vi "CPU_MEM_CIA 1.vi"(5 "read all":bool, 7 "oper":enum16{"init", "read", "write"}(ring), 10 "value in":u8 format="%02x", 11 "address":u16 format="%04x") -> (2 "value out":u8 format="%02x", 3 "mem":u8[](array[numeric])=[27, 8, 14, 6, 20] format="%02x")   [LabVIEW 2018]
uses:
  CIA/CIA_IRQ_oper.ctl
  CIA/CIA1/CIA1_glb.vi
panel:
  in  "init size":u16=255 format="%.0x"
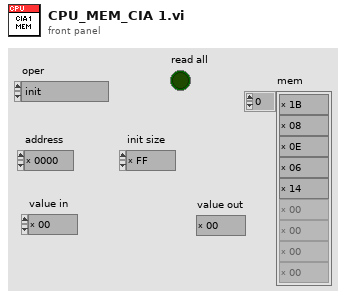
[diagram p1: front panel]
types:
  T1 = typedef "CIA_IRQ_oper.ctl" = enum16{"init", "set mask", "set flag", "check active", "read reg"}
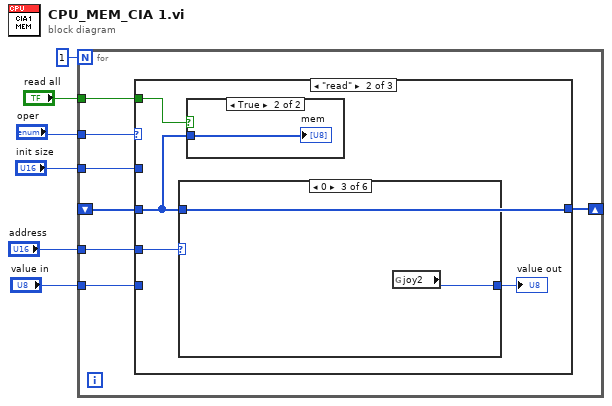
[diagram p0: block diagram]
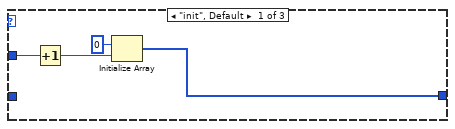
[diagram p2: hidden frame]
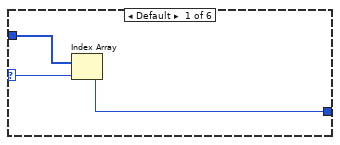
[diagram p4: hidden frame]
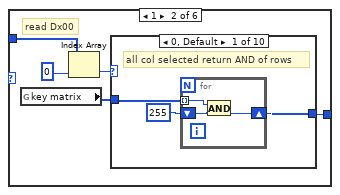
[diagram p5: hidden frame]
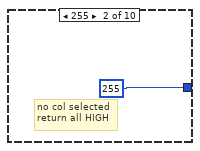
[diagram p6: hidden frame]
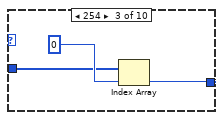
[diagram p7: hidden frame]
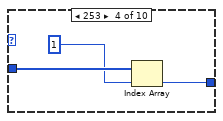
[diagram p8: hidden frame]
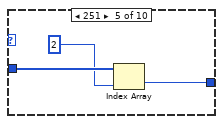
[diagram p9: hidden frame]
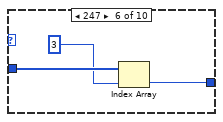
[diagram p10: hidden frame]
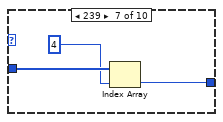
[diagram p11: hidden frame]
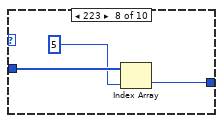
[diagram p12: hidden frame]
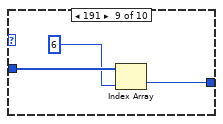
[diagram p13: hidden frame]
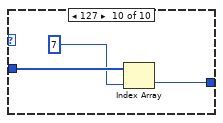
[diagram p14: hidden frame]
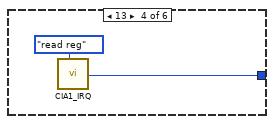
[diagram p15: hidden frame]
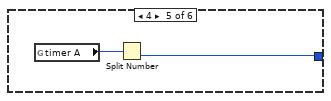
[diagram p16: hidden frame]
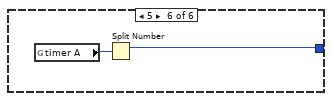
[diagram p17: hidden frame]
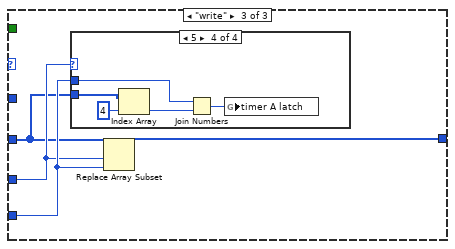
[diagram p18: hidden frame]
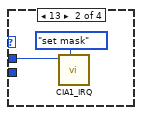
[diagram p20: hidden frame]
diagram:
  n1 = for {
    N: 1 -> [_]
    shift-right: [w11] -> _
    shift-left: _ -> [w10]
    tunnel: "oper" -> [w13]
    tunnel: "init size" -> [w12]
    tunnel: "address" -> [w9]
    tunnel: "value in" -> [w8]
    tunnel: "read all" -> [w7]
    n2 = case shown="\"read\"" w13 {
      tunnel: w12 -> [w17 _ _]
      tunnel: [w14 w19 w71] -> w11
      tunnel: w10 -> [_ w19 w69]
      tunnel: w9 -> [_ w21 w70]
      tunnel: w8 -> [_ _ w72]
      tunnel: w7 -> [_ w20 _]
      frame "init", Default {
        n3 = Increment(x=w17) -> (x+1=w15:u16)
        n4 = Initialize Array(u8 0 ("element"), w15) -> (w14:u8[])
      }
      frame "read" {
        n5 = case shown="0" w21 {
          selector: w21 -> [w23 _ _ _ _ _]
          tunnel: w19 -> [w25 w29 _ _ _ _]
          tunnel: [w24 w26 w62 w63 w65 w67] -> w18
          frame Default {
            n6 = Index Array(array=w25, index=w23) -> (element=w24:u8)
          }
          frame 1 {
            # "read Dx00"
            n7 = global read "CIA1_glb.vi" "key matrix"() -> (w30:u8[])
            n8 = Index Array(array=w29, index=0) -> (element=w28:u8)
            n9 = case shown="0, Default" w28 {
              tunnel: w30 -> [w33 _ w39 w43 w46 w49 w52 w55 w58 w61]
              tunnel: [w32 u8 255 ("y") w38 w41 w44 w47 w50 w53 w56 w59] -> w26
              frame 0, Default {
                # "all col selected return AND of rows"
                n10 = for {
                  tunnel: w33 -> [w36] mode=indexing
                  shift-right: [w34] -> w32
                  shift-left: u8 255 -> [w35]
                  n11 = And(x=w36, y=w35) -> (x .and. y?=w34:u8)
                }
              }
              frame 255 {
                # "no col selected\nreturn all HIGH"
              }
              frame 254 {
                n12 = Index Array(array=w39, index=0) -> (element=w38:u8)
              }
              frame 253 {
                n13 = Index Array(array=w43, index=1) -> (element=w41:u8)
              }
              frame 251 {
                n14 = Index Array(array=w46, index=2) -> (element=w44:u8)
              }
              frame 247 {
                n15 = Index Array(array=w49, index=3) -> (element=w47:u8)
              }
              frame 239 {
                n16 = Index Array(array=w52, index=4) -> (element=w50:u8)
              }
              frame 223 {
                n17 = Index Array(array=w55, index=5) -> (element=w53:u8)
              }
              frame 191 {
                n18 = Index Array(array=w58, index=6) -> (element=w56:u8)
              }
              frame 127 {
                n19 = Index Array(array=w61, index=7) -> (element=w59:u8)
              }
            }
          }
          frame 0 {
            n20 = global read "CIA1_glb.vi" "joy2"() -> (w62:u8)
          }
          frame 13 {
            n21 = call "CIA1_IRQ.vi"("oper"=CIA_IRQ_oper."read reg") -> ("IRQ.reg"=w63:u8)  [unwired: 9 in, 1 out]
          }
          frame 4 {
            n22 = global read "CIA1_glb.vi" "timer A"() -> (w66:u16)
            n23 = Split Number(x=w66) -> (lo(x)=w65:u8)  [unwired: 1 out]
          }
          frame 5 {
            n24 = global read "CIA1_glb.vi" "timer A"() -> (w68:u16)
            n25 = Split Number(x=w68) -> (hi(x)=w67:u8)  [unwired: 1 out]
          }
        }
        "value out" <- w18
        n26 = case shown="True" w20 {
          tunnel: w19 -> [_ w22]
          frame False {
          }
          frame True {
            "mem" <- w22
          }
        }
      }
      frame "write" {
        n27 = case shown="5" w70 {
          tunnel: w72 -> [_ w73 w76 w81]
          tunnel: w69 -> [_ _ w79 w84]
          frame Default {
          }
          frame 13 {
            n28 = call "CIA1_IRQ.vi"("oper"=CIA_IRQ_oper."set mask", "Dx0E value"=w73) -> ()  [unwired: 8 in, 2 out]
          }
          frame 4 {
            n29 = Index Array(array=w79, index=5) -> (element=w77:u8)
            n30 = Join Numbers(hi=w77, lo=w76) -> ((hi.lo)=w75:u16)
            n31 = global write "CIA1_glb.vi" "timer A latch"(w75) -> ()
          }
          frame 5 {
            n32 = Index Array(array=w84, index=4) -> (element=w82:u8)
            n33 = Join Numbers(hi=w81, lo=w82) -> ((hi.lo)=w80:u16)
            n34 = global write "CIA1_glb.vi" "timer A latch"(w80) -> ()
          }
        }
        n35 = Replace Array Subset(array=w69, new element=w72, index=w70) -> (w71:u8[])
      }
    }
  }
